vi "Initialize.vi"(8 "error in (no error)":errorcluster, 11 "SSI PR Settings In":T1={"VISA resource name"="", "Simulated?"=TRUE}) -> (0 "error out":errorcluster, 1 "Initialized":bool, 2 "No Pump Connected":bool, 3 "SSI PR Settings Out":T1={"VISA resource name"="", "Simulated?"=TRUE})   [LabVIEW 2021]
uses:
  SSI PR Settings Cluster.ctl
  <vilib>/Instr/_visa.llb/VISA Configure Serial Port (Instr).vi
panel:
  out "read buffer":string
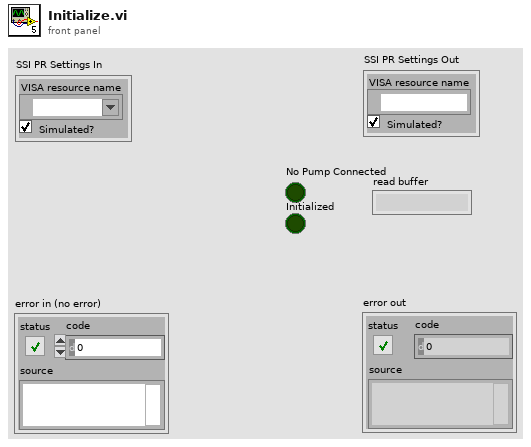
[diagram p1: front panel]
types:
  T1 = typedef "SSI PR Settings Cluster.ctl" = cluster{"VISA resource name":refnum<visa-resource-name>, "Simulated?":bool}
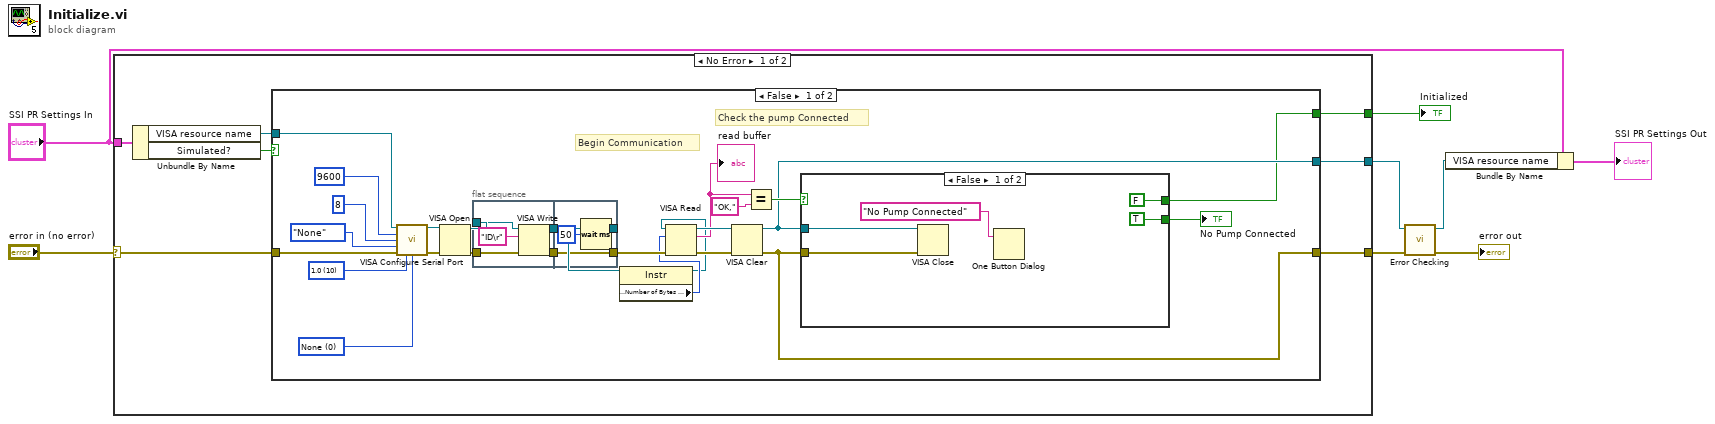
[diagram p0: block diagram]
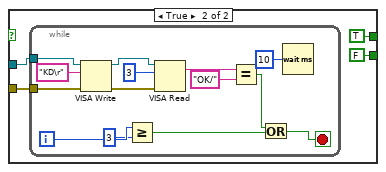
[diagram p2: hidden frame]
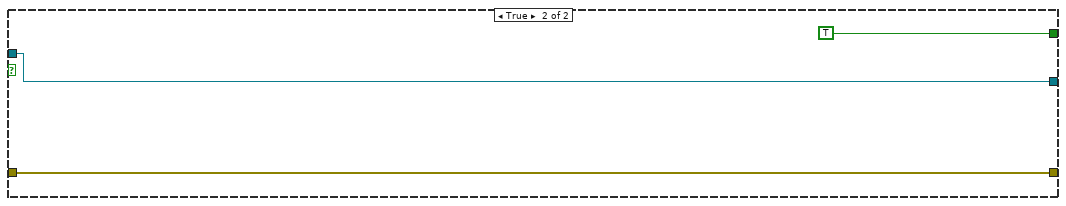
[diagram p3: hidden frame]
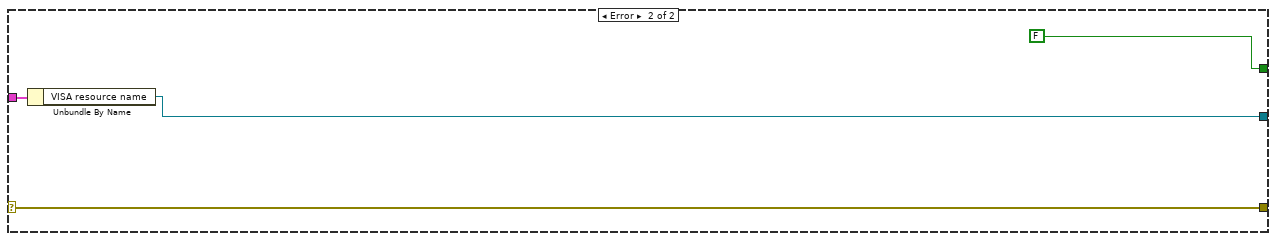
[diagram p4: hidden frame]
diagram:
  n1 = case shown="No Error" "error in (no error)" {
    selector: "error in (no error)" -> [w15 w79]
    tunnel: "SSI PR Settings In" -> [w11 w78]
    tunnel: [w12 w79] -> w5
    tunnel: [w10 w77] -> w4
    tunnel: [w9 FALSE] -> w3
    frame No Error {
      n2 = Unbundle By Name(w11) -> ("VISA resource name"=w13:refnum<visa-resource-name>, "Simulated?"=w14:bool)
      n3 = case shown="False" w14 {
        tunnel: w15 -> [w35 w75]
        tunnel: w13 -> [w33 w74]
        tunnel: [w25 w75] -> w12
        tunnel: [w24 w74] -> w10
        tunnel: [w22 TRUE] -> w9
        frame False {
          w37 = u16 0 items=["None", "XON/XOFF", "RTS/CTS", "XON/XOFF & RTS/CTS", "DTR/DSR", "XON/XOFF & DTR/DSR"] ("flow control (0:none)")
          w38 = u16 10 items=["1.0"=10, "1.5"=15, "2.0"=20] ("stop bits (10: 1 bit)")
          # "Check the pump Connected"
          # "Begin Communication"
          n4 = call-poly "VISA Configure Serial Port"("VISA resource name"=w33, "baud rate (9600)"=u32 9600, "data bits (8)"=u16 8, "parity (0:none)"=enum16{"None", "Odd", "Even", "Mark", "Space"}."None", "error in (no error)"=w35, "stop bits (10: 1 bit)"=w38, "flow control (0:none)"=w37) -> ("VISA resource name out"=w34:refnum<visa-resource-name>, "error out"=w36:errorcluster)  [unwired: 7 in]
          n5 = VISA Open(error in (no error)=w36, VISA resource name=w34) -> (VISA resource name=w32:refnum<visa-resource-name>, error out=w31:errorcluster)  [unwired: 3 in]
          n6 = flat-sequence {
            tunnel: w32 -> [w46]
            tunnel: w31 -> [w45]
            tunnel: [w43] -> w17
            tunnel: [w42] -> w16
            tunnel: [w48] -> w20
            tunnel: [w49] -> w21
            tunnel: w17 -> [w49]
            tunnel: w16 -> [w48]
            frame #0 {
              n7 = VISA Write(VISA resource name=w46, write buffer="ID\r", error in (no error)=w45) -> (VISA resource name out=w42:refnum<visa-resource-name>, error out=w43:errorcluster)  [unwired: 1 out]
            }
            frame #1 {
              n8 = Wait (ms)(milliseconds to wait=u32 50) -> ()  [unwired: 1 out]
            }
          }
          n9 = property class="Instr"(reference=w20) -> (reference out=w18:refnum<visa-resource-name>, "Serial Settings:Number of Bytes at Serial Port"=w19:u32)  [unwired: 1 in, 1 out]
          n10 = VISA Read(VISA resource name=w18, byte count=w19, error in (no error)=w21) -> (VISA resource name out=w28:refnum<visa-resource-name>, read buffer=w26:string, error out=w29:errorcluster)  [unwired: 1 out]
          "read buffer" <- w26
          n11 = VISA Clear(VISA resource name=w28, error in (no error)=w29) -> (VISA resource name out=w24:refnum<visa-resource-name>, error out=w25:errorcluster)
          n12 = Equal?(x=w26, y="OK,") -> (x = y?=w30:bool)
          n13 = case shown="False" w30 {
            tunnel: w24 -> [w53 w56]
            tunnel: w25 -> [w52 w55]
            tunnel: [TRUE FALSE] -> w23
            tunnel: [FALSE TRUE] -> w22
            frame False {
              n14 = VISA Close(VISA resource name=w53, error in (no error)=w52) -> ()  [unwired: 1 out]
              n15 = One Button Dialog(message="No Pump Connected") -> ()  [unwired: 1 in, 1 out]
            }
            frame True {
              n16 = while {
                tunnel: w56 -> [w71]
                tunnel: w55 -> [w70]
                i -> [w62]
                stop <- w63 stop-if-true
                n17 = VISA Write(VISA resource name=w71, write buffer="KD\r", error in (no error)=w70) -> (VISA resource name out=w68:refnum<visa-resource-name>, error out=w67:errorcluster)  [unwired: 1 out]
                n18 = Greater Or Equal?(x=w62, y=3) -> (x >= y?=w60:bool)
                n19 = VISA Read(VISA resource name=w68, byte count=u32 3, error in (no error)=w67) -> (read buffer=w66:string)  [unwired: 3 out]
                n20 = Equal?(x=w66, y="OK/") -> (x = y?=w64:bool)
                n21 = Or(x=w64, y=w60) -> (x .or. y?=w63:bool)
                n22 = Wait (ms)(milliseconds to wait=u32 10) -> ()  [unwired: 1 out]
              }
            }
          }
          "No Pump Connected" <- w23
        }
        frame True {
        }
      }
    }
    frame Error {
      n23 = Unbundle By Name(w78) -> ("VISA resource name"=w77:refnum<visa-resource-name>)
    }
  }
  "Initialized" <- w3
  n24 = call "Error Checking.vi"("error in (no error)"=w5, "VISA resource name"=w4) -> ("error out"=→"error out":errorcluster, "VISA resource name"=w7:refnum<visa-resource-name>)  [unwired: 7 in, 1 out]
  n25 = Bundle By Name(cluster="SSI PR Settings In", "VISA resource name"=w7) -> (→"SSI PR Settings Out":T1)
